vi "Save_to_Project.vi"(8 "error in (no error)":errorcluster, 9 "index in":string, 10 "buildObject":T2, 11 "IB_RegData_I32 in":refnum<class "IB_RegData_I32.lvclass">) -> (0 "error out":errorcluster, 1 "index out":string, 2 "buildObject out":T2, 3 "IB_RegData_I32 out":refnum<class "IB_RegData_I32.lvclass">)   [LabVIEW 2020, in "IB_RegData_I32.lvclass"]
uses:
  <vilib>/AppBuilder/IB_Classes/RegData/RegData_I32/IB_RegData_I32.lvclass
  <vilib>/AppBuilder/IB_Classes/RegData/RegData_I32/IB_RegData_I32.lvclass/IB_RegData_I32.ctl
  <vilib>/AppBuilder/IB_RW_Project/IB_RW_Project_PropBag_Action.ctl
  <vilib>/AppBuilder/IB_Classes/RegData/IB_RegData.lvclass
  <resource>/Framework/Providers/API/ItemRef.ctl
  <vilib>/AppBuilder/IB_RW_Project/IB_RW_Project_RegData_I32_Data.ctl
panel:
  in  "RegData":T1
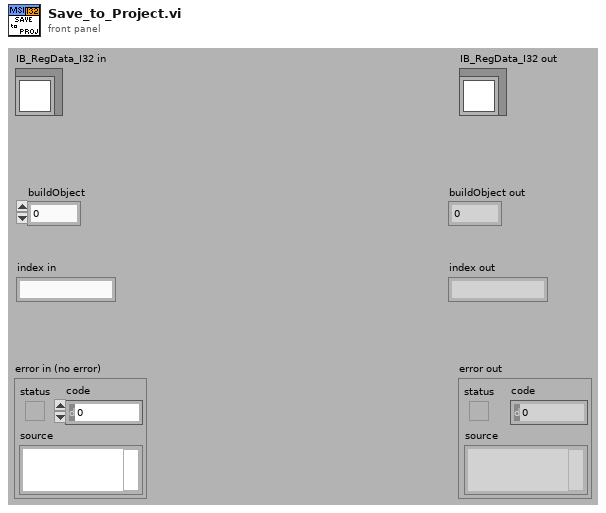
[diagram p1: front panel]
types:
  T1 = typedef "IB_RW_Project_RegData_I32_Data.ctl" = cluster{"I32":i32}
  T2 = typedef "ItemRef.ctl" = u64
  T3 = typedef "IB_RW_Project_PropBag_Action.ctl" = enum16{"read", "write", "clear", "readPrevious", "writePrevious", "clearPrevious"}
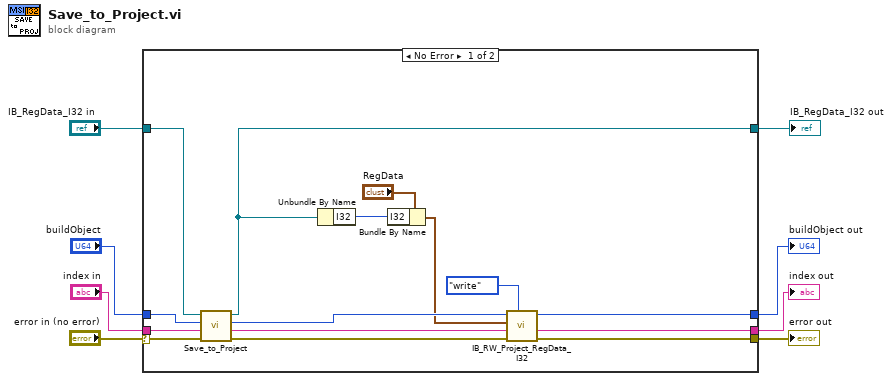
[diagram p0: block diagram]
diagram:
  n1 = case shown="No Error" "error in (no error)" {
    selector: "error in (no error)" -> [w20 w27]
    tunnel: [w17 w27] -> w8
    tunnel: [w15 w26] -> w7
    tunnel: [w13 w25] -> w6
    tunnel: [w19 w24] -> w5
    tunnel: "index in" -> [w23 w26]
    tunnel: "buildObject" -> [w22 w25]
    tunnel: "IB_RegData_I32 in" -> [w21 w24]
    frame No Error {
      n2 = call-parent "Save_to_Project.vi"("error in (no error)"=w20, "index in"=w23, "buildObject"=w22, "IB_RegData in"=w21) -> ("error out"=w18:errorcluster, "index out"=w16:string, "buildObject out"=w14:T2, "IB_RegData out"=w19:refnum<class "IB_RegData_I32.lvclass">)  [unwired: 4 in]
      n3 = Unbundle By Name(w19) -> ("I32"=w10:i32)
      n4 = Bundle By Name(cluster="RegData", "I32"=w10) -> (w9:T1)
      n5 = call <vilib>:"IB_RW_Project_RegData_I32.vi"("action"=IB_RW_Project_PropBag_Action."write", "error in (no error)"=w18, "index in"=w16, "RegData"=w9, "buildObject"=w14) -> ("error out"=w17:errorcluster, "index out"=w15:string, "buildObject out"=w13:T2)  [unwired: 3 in, 1 out]
    }
    frame Error {
    }
  }
  "error out" <- w8
  "IB_RegData_I32 out" <- w5
  "buildObject out" <- w6
  "index out" <- w7
